vi "Get All Controls and Indicators.vi"(0 "controls[]":refnum<vi>[](array[refnum]), 11 "error in":errorcluster) -> (4 "controls[]":refnum<vi>[](array[refnum]), 6 "indicators[]":refnum<vi>[](array[refnum]), 15 "error out":errorcluster)   [LabVIEW 2021, in "Converter.lvlib"]
uses:
  Converter.lvlib
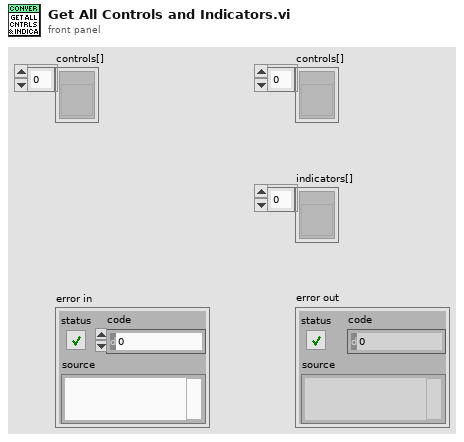
[diagram p1: front panel]
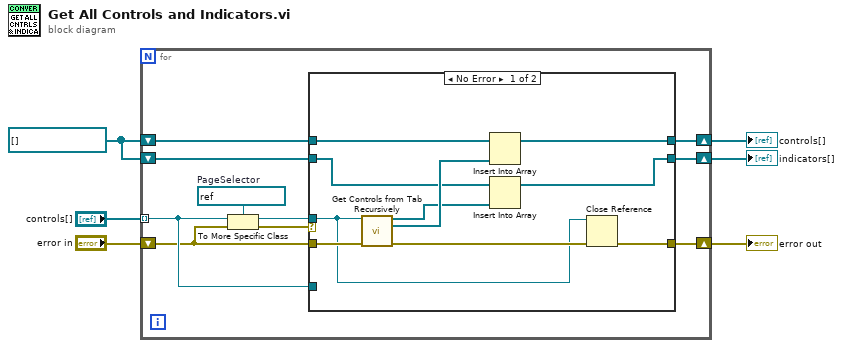
[diagram p0: block diagram]
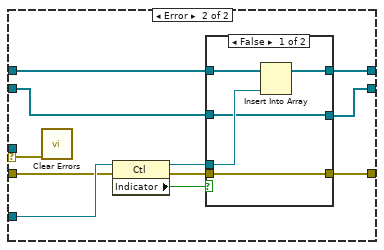
[diagram p2: hidden frame]
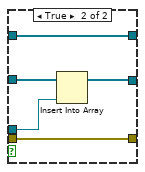
[diagram p3: hidden frame]
diagram:
  w3 = refnum<vi>[] []
  n1 = for {
    tunnel: "controls[]" -> [w13] mode=indexing
    shift-right: [w9] -> w4
    shift-left: w3 -> [w12]
    shift-right: [w10] -> w5
    shift-left: w3 -> [w11]
    shift-right: [w7] -> w2
    shift-left: "error in" -> [w8]
    w16 = refnum<vi> refnum  # PageSelector
    n2 = To More Specific Class(target class=w16, reference=w13, error in=w8) -> (specific class reference=w14:refnum<vi>, error out=w15:errorcluster)
    n3 = case shown="No Error" w15 {
      selector: w15 -> [_ w28]
      tunnel: w14 -> [w18 _]
      tunnel: w13 -> [_ w35]
      tunnel: w12 -> [w23 w36]
      tunnel: w11 -> [w25 w37]
      tunnel: [w24 w32] -> w10
      tunnel: [w22 w33] -> w9
      tunnel: w8 -> [w21 w30]
      tunnel: [w19 w29] -> w7
      frame No Error {
        n4 = call "Get Controls from Tab Recursively.vi"("page sel refnum"=w18, "error in"=w21) -> ("indicators in tab"=w17:refnum<vi>[], "controls in tab"=w26:refnum<vi>[], "error out"=w20:errorcluster)  [unwired: 11 in]
        n5 = Insert Into Array(array=w25, new element=w26) -> (w24:refnum<vi>[])  [unwired: 1 in]
        n6 = Insert Into Array(array=w23, new element=w17) -> (w22:refnum<vi>[])  [unwired: 1 in]
        n7 = Close Reference(reference=w18, error in (no error)=w20) -> (error out=w19:errorcluster)
      }
      frame Error {
        n8 = call <vilib>:"Clear Errors.vi"("error in (no error)"=w28) -> ()  [unwired: 5 in, 2 out]
        n9 = property class="Ctl"(reference=w35, error in=w30) -> (reference out=w34:refnum<vi>, error out=w31:errorcluster, "Indicator"=w27:bool)
        n10 = case shown="False" w27 {
          tunnel: w37 -> [w38 w44]
          tunnel: w36 -> [w41 w47]
          tunnel: w34 -> [w42 w46]
          tunnel: [w41 w45] -> w33
          tunnel: [w39 w44] -> w32
          tunnel: w31 -> [w40 w43]
          tunnel: [w40 w43] -> w29
          frame False {
            n11 = Insert Into Array(array=w38, new element=w42) -> (w39:refnum<vi>[])  [unwired: 1 in]
          }
          frame True {
            n12 = Insert Into Array(array=w47, new element=w46) -> (w45:refnum<vi>[])  [unwired: 1 in]
          }
        }
      }
    }
  }
  "controls[]" <- w5
  "indicators[]" <- w4
  "error out" <- w2
